vi "OPC UA Server2.vi"() -> ()   [LabVIEW 2017]
uses:
  <vilib>/OPCUA/controls/NodeId.ctl
  <vilib>/OPCUA/controls/Data Type.ctl
  <vilib>/OPCUA/server/Write Int32.vi
  <vilib>/OPCUA/server/Read Int32.vi
  <vilib>/OPCUA/NI OPC UA Server.lvlib
panel:
  out "value 2":i32
  out "value":i32
  out "item node ID":T1
  out "server endpoint URL":string
  out "error out":errorcluster
  in  "stop":bool
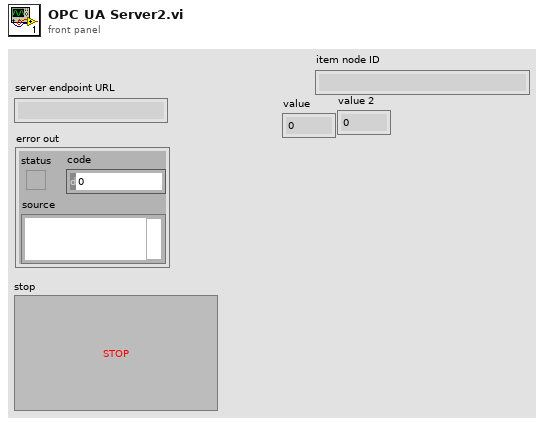
[diagram p1: front panel]
types:
  T1 = typedef "NodeId.ctl" = string
  T2 = typedef "Data Type.ctl" = u16
  T3 = cluster{"name":string, "data type":T2, "access level":u16, "description":string}
  T4 = typedef "OPC UA Server Refnum.ctl" = refnum<k21>
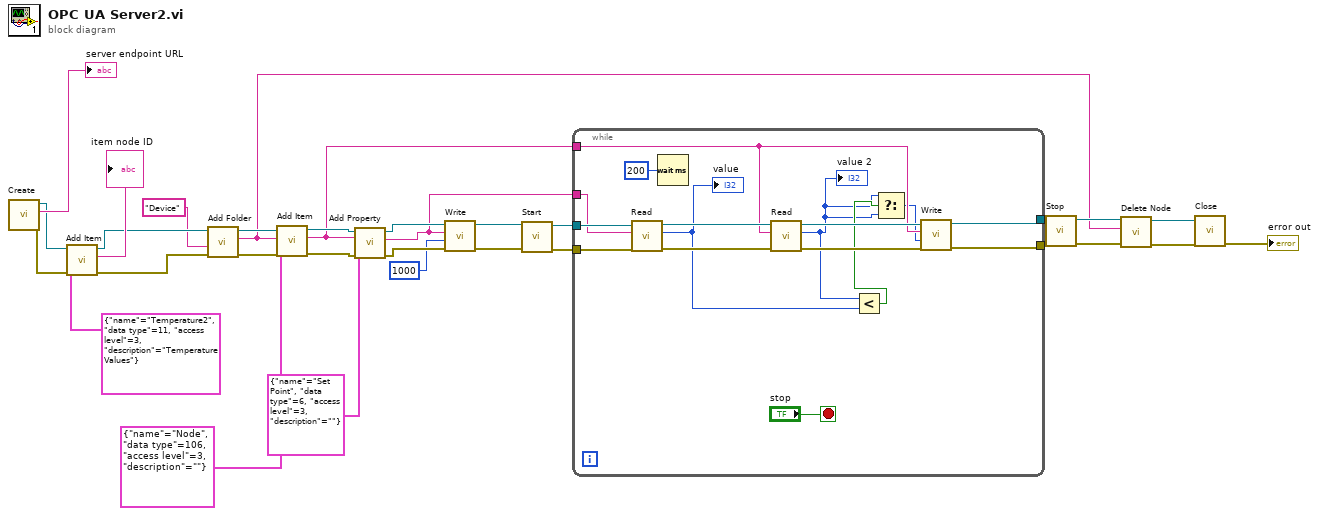
[diagram p0: block diagram]
diagram:
  n1 = call <vilib>:"Create.vi"() -> ("error out"=w26:errorcluster, "server endpoint URL"=→"server endpoint URL":string, "OPC UA server refnum out"=w27:T4)  [unwired: 9 in]
  n2 = call <vilib>:"Add Item.vi"("error in (no error)"=w26, "item"=T3 {"name"="Temperature2", "data type"=11, "access level"=3, "description"="Temperature Values"}, "OPC UA server refnum in"=w27) -> ("error out"=w10:errorcluster, "item node ID"=→"item node ID":T1, "OPC UA server refnum out"=w11:T4)  [unwired: 4 in, 1 out]
  n3 = call <vilib>:"Add Folder.vi"("error in (no error)"=w10, "folder name"="Device", "OPC UA server refnum in"=w11) -> ("error out"=w12:errorcluster, "folder node ID"=w3:T1, "OPC UA server refnum out"=w13:T4)  [unwired: 5 in]
  n4 = call <vilib>:"Add Item.vi"("error in (no error)"=w12, "item"=T3 {"name"="Node", "data type"=106, "access level"=3, "description"=""}, "parent folder node ID"=w3, "OPC UA server refnum in"=w13) -> ("error out"=w22:errorcluster, "item node ID"=w1:T1, "OPC UA server refnum out"=w2:T4)  [unwired: 3 in, 1 out]
  n5 = call <vilib>:"Add Property.vi"("error in (no error)"=w22, "property"=T3 {"name"="Set Point", "data type"=6, "access level"=3, "description"=""}, "item node ID"=w1, "OPC UA server refnum in"=w2) -> ("error out"=w18:errorcluster, "property node ID"=w14:T1, "OPC UA server refnum out"=w20:T4)  [unwired: 3 in, 1 out]
  n6 = call-poly <vilib>:"Write.vi"("error in (no error)"=w18, "value"=1000, "node ID"=w14, "OPC UA server refnum in"=w20) -> ("error out"=w17:errorcluster, "OPC UA server refnum out"=w19:T4)  [unwired: 5 in, 1 out]
  n7 = call <vilib>:"Start.vi"("error in (no error)"=w17, "OPC UA server refnum in"=w19) -> ("error out"=w15:errorcluster, "OPC UA server refnum out"=w16:T4)  [unwired: 7 in, 1 out]
  n8 = while {
    tunnel: [w43] -> w31
    tunnel: [w42] -> w30
    tunnel: w16 -> [w45]
    tunnel: w15 -> [w44]
    tunnel: w14 -> [w41]
    tunnel: w1 -> [w36]
    stop <- "stop" stop-if-true
    n9 = call-poly <vilib>:"Read.vi"("error in (no error)"=w44, "node ID"=w41, "OPC UA server refnum in"=w45) -> ("error out"=w39:errorcluster, "value"=w35:i32, "OPC UA server refnum out"=w40:T4)  [unwired: 4 in, 2 out]
    "value" <- w35
    n10 = Wait (ms)(milliseconds to wait=u32 200) -> ()  [unwired: 1 out]
    n11 = call-poly <vilib>:"Read.vi"("error in (no error)"=w39, "node ID"=w36, "OPC UA server refnum in"=w40) -> ("error out"=w37:errorcluster, "value"=w33:i32, "OPC UA server refnum out"=w38:T4)  [unwired: 4 in, 2 out]
    "value 2" <- w33
    n12 = Less?(x=w33, y=w35) -> (x < y?=w34:bool)
    n13 = Select(t=w33, s=w34, f=w33) -> (s? t:f=w32:i32)
    n14 = call-poly <vilib>:"Write.vi"("error in (no error)"=w37, "value"=w32, "node ID"=w36, "OPC UA server refnum in"=w38) -> ("error out"=w42:errorcluster, "OPC UA server refnum out"=w43:T4)  [unwired: 5 in, 1 out]
  }
  n15 = call <vilib>:"Stop.vi"("error in (no error)"=w30, "OPC UA server refnum in"=w31) -> ("error out"=w5:errorcluster, "OPC UA server refnum out"=w7:T4)  [unwired: 8 in]
  n16 = call <vilib>:"Delete Node.vi"("error in (no error)"=w5, "node ID"=w3, "OPC UA server refnum in"=w7) -> ("error out"=w4:errorcluster, "OPC UA server refnum out"=w6:T4)  [unwired: 7 in]
  n17 = call <vilib>:"Close.vi"("error in (no error)"=w4, "OPC UA server refnum in"=w6) -> ("error out"=→"error out":errorcluster)  [unwired: 9 in]
